vi "nti.vi"(11 "Number to match":u32) -> (2 "Iterations":u32, 3 "Time to match, s":dbl)   [LabVIEW 2024]
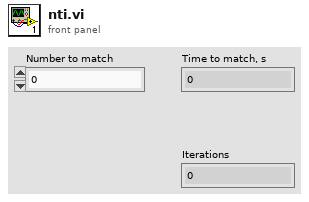
[diagram p1: front panel]
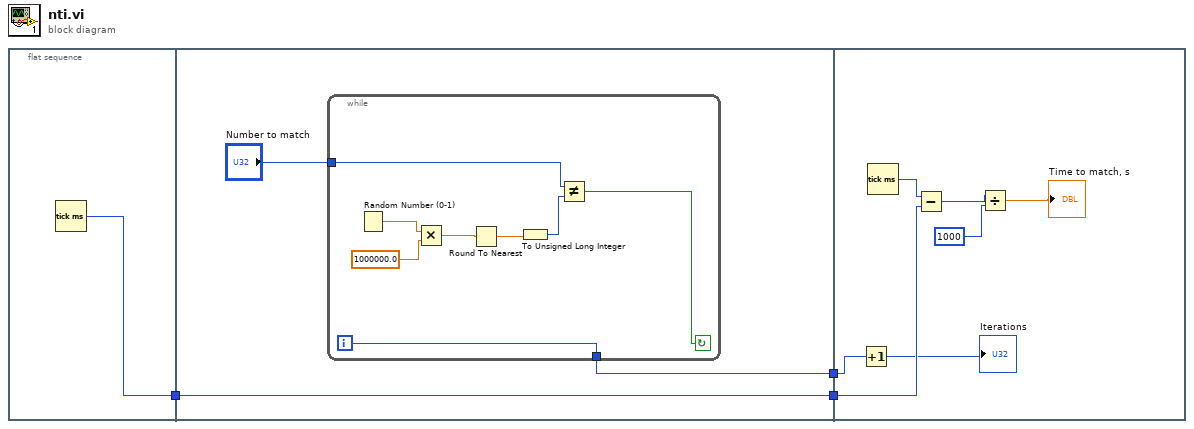
[diagram p0: block diagram]
diagram:
  n1 = flat-sequence {
    tunnel: [w4] -> w3
    tunnel: [w6] -> w2
    tunnel: w3 -> [w5]
    tunnel: [w5] -> w1
    tunnel: w2 -> [w17]
    tunnel: w1 -> [w21]
    frame #0 {
      n2 = Tick Count (ms)() -> (millisecond timer value=w4:u32)
    }
    frame #1 {
      n3 = while {
        tunnel: "Number to match" -> [w11]
        tunnel: [w10] -> w6
        i -> [w10]
        stop <- w9 continue-if-true
        n4 = Random Number (0-1)() -> (number: 0 to 1=w15:dbl)
        n5 = Multiply(x=w15, y=1000000.0) -> (x*y=w14:dbl)
        n6 = Round To Nearest(number=w14) -> (nearest integer value=w13:dbl)
        n7 = To Unsigned Long Integer(number=w13) -> (unsigned 32bit integer=w12:u32)
        n8 = Not Equal?(x=w11, y=w12) -> (x != y?=w9:bool)
      }
    }
    frame #2 {
      n9 = Increment(x=w17) -> (x+1=→"Iterations":i32)
      n10 = Tick Count (ms)() -> (millisecond timer value=w22:u32)
      n11 = Subtract(x=w22, y=w21) -> (x-y=w19:u32)
      n12 = Divide(x=w19, y=1000) -> (x/y=→"Time to match, s":dbl)
    }
  }
